vi "BooleanToTrueFalseEnumvi.vi"(11 "selection":bool) -> (3 "On/Off":enum16{"off", "on"}(ring))   [LabVIEW 2020]
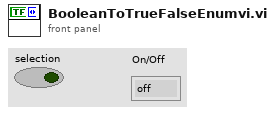
[diagram p1: front panel]
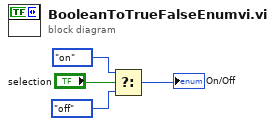
[diagram p0: block diagram]
diagram:
  n1 = Select(t=enum16{"off", "on"}."on" ("ChannelOn"), s="selection", f=enum16{"off", "on"}."off" ("ChannelOn")) -> (s? t:f=→"On/Off":enum16{"off", "on"})
